vi "Stall Detection.vi"(11 "NXT/EV3":T1) -> (3 "NXT/EV3":T1)   [LabVIEW 2016]
uses:
  <vilib>/NXT/Subs/LVHSConnector.ctl
  <vilib>/NXT/LegoClasses/BrickReference/BrickReference.lvclass
  <vilib>/NXT/Block Support/NXT_OutputPort.ctl
  <vilib>/NXT/Block Support/NXT_TimerIndex.ctl
  <vilib>/NXT/NXTIO Xnodes/NXTIONodeSubVIs/NXTMoveMotors.vi
  <vilib>/NXT/NXTIO Xnodes/NXTIONodeSubVIs/LEGOResetMotors.vi
  <vilib>/NXT/Dual Mode Library/Sensors/Reset_Timer.vi
  <vilib>/NXT/Dual Mode Library/Waits/Wait_Num.vi
  <vilib>/NXT/Dual Mode Library/Motors/Rotation.vi
  <vilib>/NXT/Dual Mode Library/Sensors/Read_Timer.vi
  <vilib>/NXT/NXTIO Xnodes/NXTIONodeSubVIs/NXTStopMotors.vi
  <vilib>/NXT/NXTIO Xnodes/NXTIOXNode/NXTIO.xnode
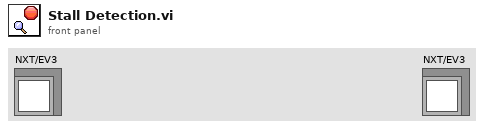
[diagram p1: front panel]
types:
  T1 = typedef "LVHSConnector.ctl" = refnum<class "BrickReference.lvclass">
  T2 = typedef "NXT_OutputPort.ctl" = u8
  T3 = typedef "NXT_TimerIndex.ctl" = u8
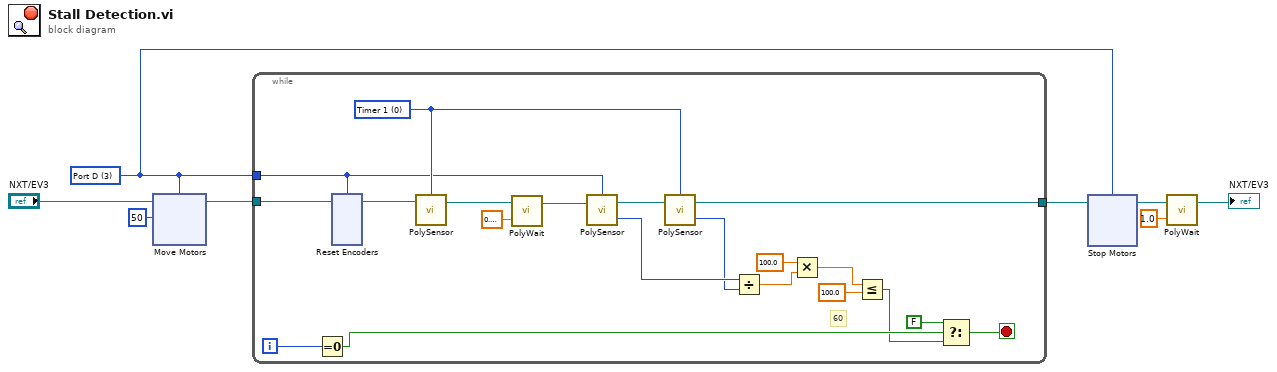
[diagram p0: block diagram]
diagram:
  w5 = T2 3 items=["Port A", "Port B", "Port C", "Port D"] ("Port (Port A)")
  n1 = xnode "Move Motors"("Power/Speed 1"=i8 50, "Motors"=w5, "NXT/EV3"="NXT/EV3") -> ("NXT/EV3"=w8:T1)
  n2 = while {
    tunnel: w8 -> [w20]
    tunnel: [w19] -> w6
    tunnel: w5 -> [w18]
    i -> [w13]
    stop <- w10 stop-if-true
    w24 = T3 0 items=["Timer 1", "Timer 2", "Timer 3"] ("Timer (Timer 1)")
    # "60"
    n3 = Equal To 0?(x=w13) -> (x = 0?=w12:bool)
    n4 = xnode "Reset Encoders"("Motors"=w18, "NXT/EV3"=w20) -> ("NXT/EV3"=w28:T1)
    n5 = call-poly <vilib>:"PolySensor.vi"("NXT/EV3"=w28, "Timer (Timer 1)"=w24) -> ("NXT/EV3"=w27:T1)  [unwired: 2 in]
    n6 = call-poly <vilib>:"PolyWait.vi"("Time (1 sec)"=sgl 0.2, "NXT/EV3"=w27) -> ("NXT/EV3"=w25:T1)  [unwired: 2 in]
    n7 = call-poly <vilib>:"PolySensor.vi"("NXT/EV3"=w25, "Port (Port A)"=w18) -> ("Angle of Rotation"=w22:i32, "NXT/EV3"=w23:T1)  [unwired: 1 in]
    n8 = call-poly <vilib>:"PolySensor.vi"("NXT/EV3"=w23, "Timer (Timer 1)"=w24) -> ("Value (msec)"=w21:u32, "NXT/EV3"=w19:T1)  [unwired: 1 in]
    n9 = Divide(x=w22, y=w21) -> (x/y=w16:dbl)
    n10 = Multiply(x=100.0 ("y"), y=w16) -> (x*y=w15:dbl)
    n11 = Less Or Equal?(x=w15, y=100.0) -> (x <= y?=w9:bool)
    n12 = Select(t=FALSE, s=w12, f=w9) -> (s? t:f=w10:bool)
  }
  n13 = xnode "Stop Motors"("Motors"=w5, "NXT/EV3"=w6) -> ("NXT/EV3"=w3:T1)
  n14 = call-poly <vilib>:"PolyWait.vi"("Time (1 sec)"=sgl 1.0, "NXT/EV3"=w3) -> ("NXT/EV3"=→"NXT/EV3":T1)  [unwired: 2 in]
